vi "Controlador_DAQ_PID.vi"() -> ()   [LabVIEW 2012]
panel:
  in  "Velocidad deseada\nRPM":dbl
  out "control ant":dbl
  out "error ant":dbl
  out "error":dbl
  out "Waveform Chart 2":dbl(graph)
  in  "stop":bool
  out "Waveform Chart":dbl(graph)
  in  "u_ini":dbl
  in  "error_ini":dbl
  # "MAX 3000"
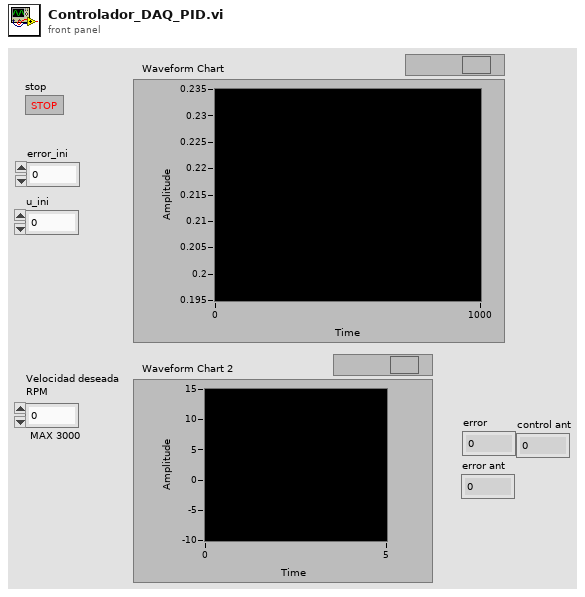
[diagram p1: front panel]
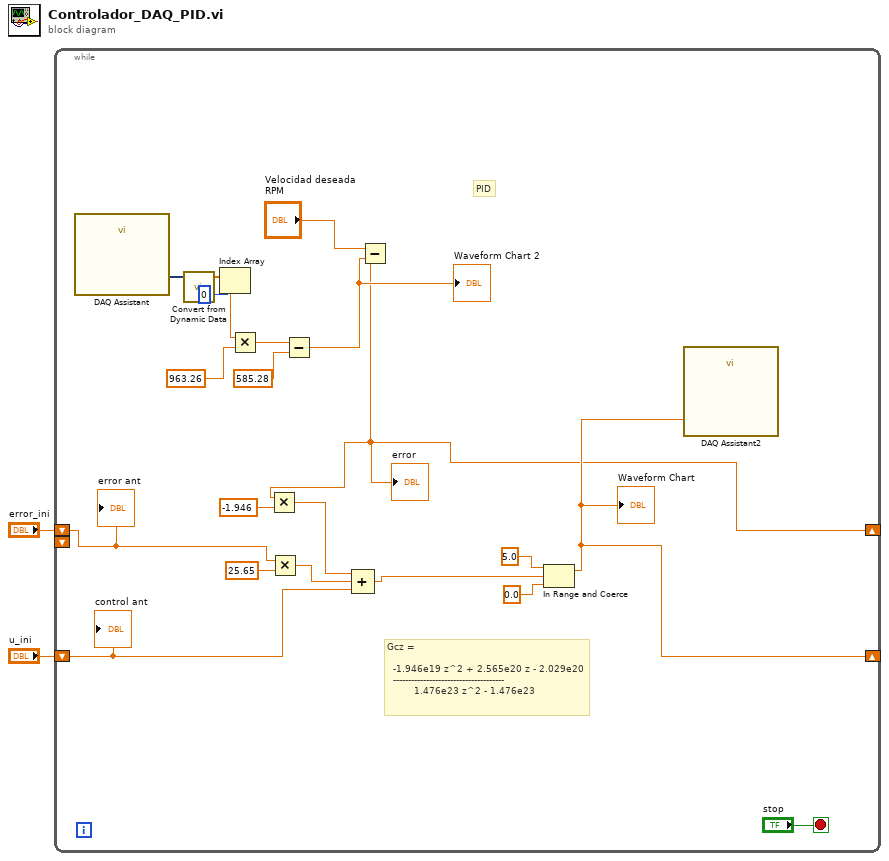
[diagram p0: block diagram]
diagram:
  n1 = while {
    shift-right: [w4] -> _
    shift-left: "error_ini" -> [w19]
    shift-right: [w9] -> _
    shift-left: "u_ini" -> [w18]
    shift-left: _ -> [_]
    stop <- "stop" stop-if-true
    # "Gcz =\n \n  -1.946e19 z^2 + 2.565e20 z - 2.029e20\n  -------------------------------------\n         1.476e23 z^2 - 1.476e23"
    # "PID"
    n2 = call "DAQ Assistant"() -> ("data"=w6:dynamicdata)  [unwired: 17 in, 2 out]
    n3 = call "Convert from Dynamic Data"("Dynamic Data Type"=w6) -> ("Array"=w11:dbl[])  [unwired: 3 in]
    n4 = Index Array(array=w11, index=0) -> (element=w5:dbl)
    n5 = Multiply(x=w5, y=963.26) -> (x*y=w16:dbl)
    n6 = Multiply(x=w19, y=25.65) -> (x*y=w23:dbl)
    n7 = Subtract(x=w16, y=585.28) -> (x-y=w7:dbl)
    "Waveform Chart 2" <- w7
    n8 = Subtract(x="Velocidad deseada\nRPM", y=w7) -> (x-y=w4:dbl)
    "error" <- w4
    n9 = Multiply(x=w4, y=-1.946) -> (x*y=w22:dbl)
    n10 = Compound Arithmetic op=ADD(w22, w23, w18) -> (w14:dbl)
    n11 = In Range and Coerce(upper limit=5.0, x=w14, lower limit=0.0) -> (coerced(x)=w9:dbl)  [unwired: 1 out]
    "Waveform Chart" <- w9
    n12 = call "DAQ Assistant2"("data"=w9) -> ()  [unwired: 17 in, 2 out]
    "error ant" <- w19
    "control ant" <- w18
  }
